vi "PV Set Pressure Data.vi"(1 "Pressure (mbar)\n0 ==> ur (<1,0e-4mbar)\n1 - 2050 mbar":i16 min=0 max=2050 step=1) -> (0 "Output":string)   [LabVIEW 2016, in "Pfeiffer Vacuum.lvlib"]
uses:
  Pfeiffer Vacuum.lvlib
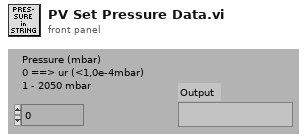
[diagram p1: front panel]
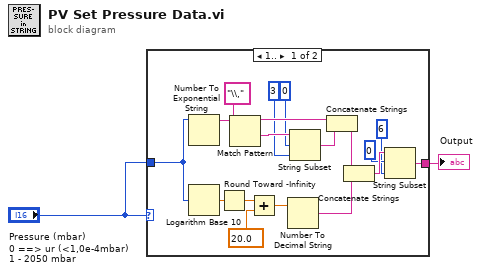
[diagram p0: block diagram]
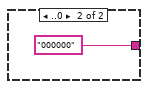
[diagram p2: hidden frame]
diagram:
  n1 = case shown="1.." "Pressure (mbar)\n0 ==> ur (<1,0e-4mbar)\n1 - 2050 mbar" {
    tunnel: [w7 "000000"] -> w2
    tunnel: "Pressure (mbar)\n0 ==> ur (<1,0e-4mbar)\n1 - 2050 mbar" -> [w3 _]
    frame 1.. {
      n2 = Number To Exponential String(number=w3) -> (E-format string=w16:string)  [unwired: 3 in]
      n3 = Logarithm Base 10(1:w3) -> (0:w20:dbl)
      n4 = Round Toward -Infinity(1:w20) -> (0:w19:dbl)
      n5 = Match Pattern(string=w16, regular expression="\\,") -> (before substring=w17:string, after substring=w15:string)  [unwired: 1 in, 2 out]
      n6 = Add(x=w19, y=20.0) -> (x+y=w11:dbl)
      n7 = Number To Decimal String(number=w11) -> (decimal integer string=w8:string)  [unwired: 1 in]
      n8 = String Subset(string=w15, offset (0)=0 ("Offset (0)"), length (rest)=3 ("Länge")) -> (substring=w12:string)
      n9 = Concatenate Strings(w17, w12) -> (w9:string)
      n10 = Concatenate Strings(w9, w8) -> (w6:string)
      n11 = String Subset(string=w6, offset (0)=0 ("Offset (0)"), length (rest)=6 ("Länge")) -> (substring=w7:string)
    }
    frame ..0 {
    }
  }
  "Output" <- w2
